vi "readStadisticDataInStadisticTable.vi"(8 "error in":errorcluster, 11 "dataToQueryOfRead":T2) -> (0 "error out":errorcluster, 3 "ClusterFormat":T1)   [LabVIEW 2014]
uses:
  <vilib>/addons/database/Connection.llb/DB Tools Open Connec (String).vi
  <vilib>/addons/database/Auxilliary.llb/DB Tools Format Datetime String (Time Stamp).vi
  <vilib>/addons/database/NI_Database_API.lvlib
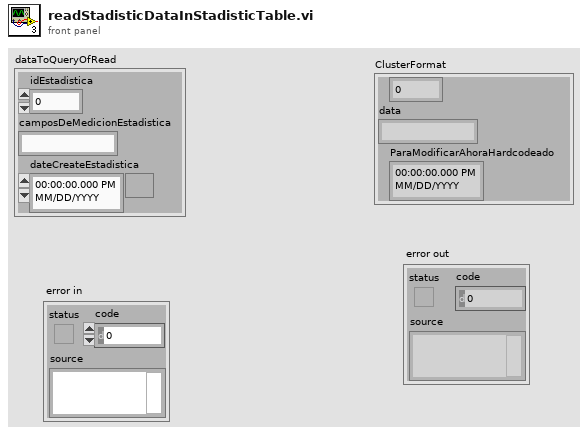
[diagram p1: front panel]
types:
  T1 = cluster{dbl, "data":string, "ParaModificarAhoraHardcodeado":timestamp}
  T2 = cluster{"idEstadistica":dbl, "camposDeMedicionEstadistica":string, "dateCreateEstadistica":timestamp}
  T3 = typedef "NI_Database_API.lvlib/Conn ObjectReference.ctl" = refnum<k1>
  T4 = typedef "NI_Database_API.lvlib/DB Tools DataTypes.ctl" = enum16{"String", "Long (I32)", "Single (SGL)", "Double (DBL)", "Date/Time", "Binary"}
  T5 = cluster{"name":string, "database data type":T4, "defined size":i32}[]
  T6 = cluster{string, "camposDeMedicionEstadistica":string, "date/time string":string}
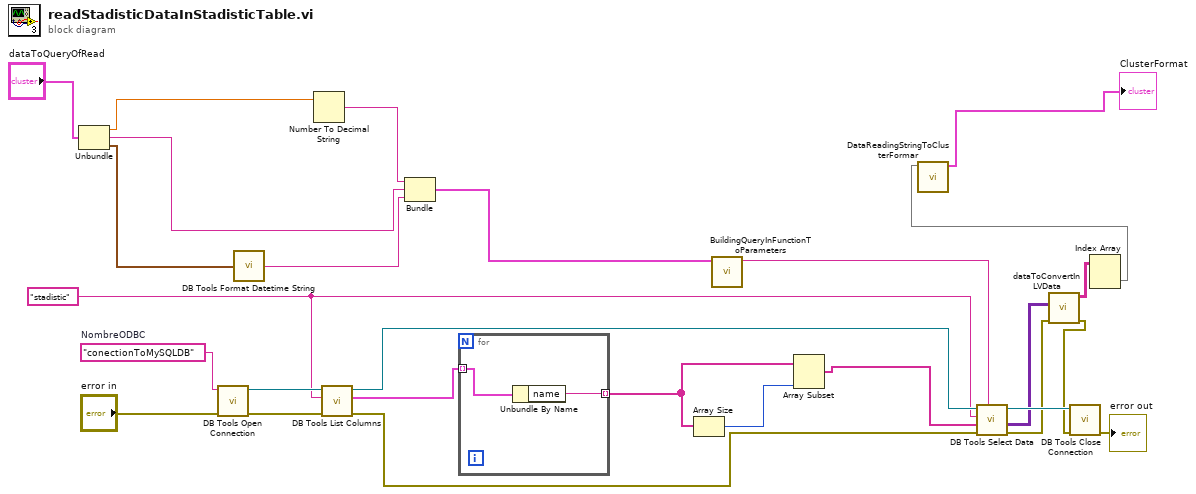
[diagram p0: block diagram]
diagram:
  w12 = "stadistic" ("tableName")
  w27 = "conectionToMySQLDB"  # NombreODBC
  n1 = Unbundle("dataToQueryOfRead") -> ("idEstadistica"=w20:dbl, "camposDeMedicionEstadistica"=w19:string, "dateCreateEstadistica"=w18:timestamp)
  n2 = call-poly <vilib>:"DB Tools Open Connection.vi"("error in (no error)"="error in", "connection information"=w27) -> ("error out"=w25:errorcluster, "connection reference"=w26:T3)  [unwired: 6 in]
  n3 = call-poly <vilib>:"DB Tools Format Datetime String.vi"("time stamp"=w18) -> ("date/time string"=w21:string)
  n4 = Number To Decimal String(number=w20) -> (decimal integer string=w22:string)  [unwired: 1 in]
  n5 = call <vilib>:"DB Tools List Columns.vi"("error in (no error)"=w25, "table"=w12, "connection reference"=w26) -> ("error out"=w13:errorcluster, "column information"=w23:T5, "connection reference out"=w14:T3)  [unwired: 1 in, 1 out]
  n6 = Bundle(w22, "camposDeMedicionEstadistica"=w19, "date/time string"=w21) -> (w11:T6)  [unwired: 1 in]
  n7 = for {
    tunnel: w23 -> [w29] mode=indexing
    tunnel: [w28] -> w16 mode=indexing
    n8 = Unbundle By Name(w29) -> ("name"=w28:string)
  }
  n9 = Array Size(array=w16) -> (size(s)=w17:i32)
  n10 = call "BuildingQueryInFunctionToParameters.vi"("ParameterToRead"=w11) -> ("QueryToRead"=w10:string)  [unwired: 10 in]
  n11 = Array Subset(array=w16, length=w17) -> (w15:string[])  [unwired: 1 in]
  n12 = call <vilib>:"DB Tools Select Data.vi"("condition"=w10, "error in (no error)"=w13, "columns"=w15, "table"=w12, "connection reference"=w14) -> ("error out"=w6:errorcluster, "data"=w7:variant[][], "connection reference out"=w9:T3)  [unwired: 1 in]
  n13 = call "dataToConvertInLVData.vi"("error in"=w6, "dataReadingIn"=w7) -> ("error out"=w5:errorcluster, "dataReadingOut"=w4:string[][])  [unwired: 8 in]
  n14 = call <vilib>:"DB Tools Close Connection.vi"("error in (no error)"=w5, "connection reference"=w9) -> ("error out"=→"error out":errorcluster)  [unwired: 5 in]
  n15 = Index Array(array=w4) -> (element=w3:string[])  [unwired: 2 in]
  n16 = call "DataReadingStringToClusterFormar.vi"("StringFormat"=w3) -> ("ClusterFormat"=→"ClusterFormat":T1)  [unwired: 10 in]
